vi "Toggle Virtual Numpad.vi"(8 "error in (no error)":errorcluster) -> (0 "error out":errorcluster)   [LabVIEW 2015, in "Utility.lvlib"]
uses:
  Utility.lvlib
  USER32.DLL
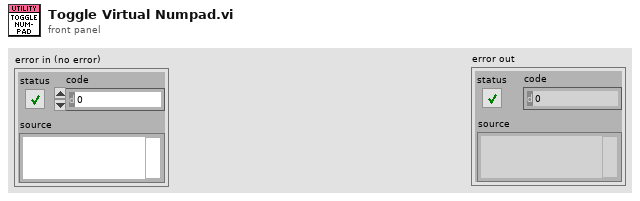
[diagram p1: front panel]
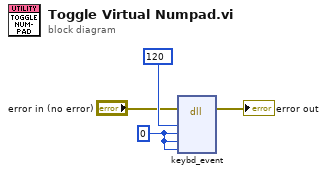
[diagram p0: block diagram]
diagram:
  w3 = u8 0 ("bScan")
  n1 = dll-call lib="user32.dll" fn="keybd_event"(error in="error in (no error)", "bVk"=u8 120 ("Virtual Key"), "bScan"=w3, "dwFlags"=w3, "dwExtraInfo"=w3) -> (error out=→"error out":errorcluster)  [unwired: 7 in, 1 out]
